vi "Read System Status.vi"(8 "error in (no error)":errorcluster) -> (0 "error out":errorcluster)   [LabVIEW 2018, in "cetoni.lvlib" / "cetoni.lvclass"]
uses:
  cetoni.lvclass
  Resources/GLOBAL/GLOBAL Time-critical.vi
  <userlib>/QmixLib/QmixLib.lvlib
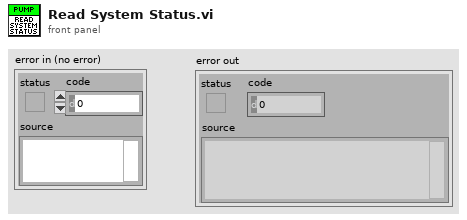
[diagram p1: front panel]
types:
  T1 = enum16{"LOW_PRESSURE_VALVE", "BALL_VALVE", "QMIX_VALVE"}
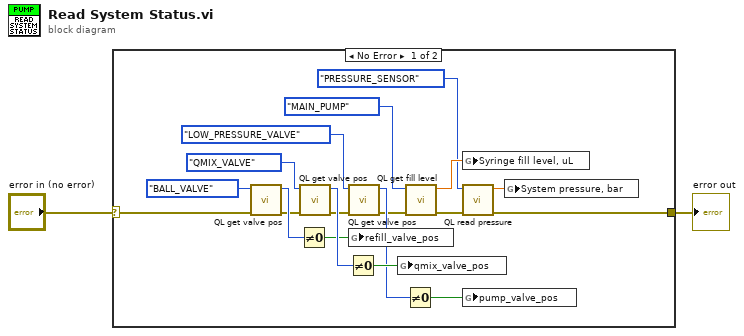
[diagram p0: block diagram]
diagram:
  n1 = case shown="No Error" "error in (no error)" {
    selector: "error in (no error)" -> [w12 w22]
    tunnel: [w5 w22] -> w1
    frame No Error {
      n2 = call <userlib>:"QL get valve pos.vi"("error in (no error) 2"=w12, "valve"=T1."BALL_VALVE") -> ("error out 2"=w11:errorcluster, "pos"=w14:i32)  [unwired: 8 in]
      n3 = Not Equal To 0?(x=w14) -> (x != 0?=w13:bool)
      n4 = call <userlib>:"QL get valve pos.vi"("error in (no error) 2"=w11, "valve"=T1."QMIX_VALVE") -> ("error out 2"=w10:errorcluster, "pos"=w19:i32)  [unwired: 8 in]
      n5 = Not Equal To 0?(x=w19) -> (x != 0?=w18:bool)
      n6 = call <userlib>:"QL get valve pos.vi"("error in (no error) 2"=w10, "valve"=T1."LOW_PRESSURE_VALVE") -> ("error out 2"=w9:errorcluster, "pos"=w16:i32)  [unwired: 8 in]
      n7 = global write "GLOBAL Time-critical.vi" "refill_valve_pos"(w13) -> ()
      n8 = global write "GLOBAL Time-critical.vi" "qmix_valve_pos"(w18) -> ()
      n9 = Not Equal To 0?(x=w16) -> (x != 0?=w15:bool)
      n10 = call <userlib>:"QL get fill level.vi"("error in (no error)"=w9, "pump"=enum16{"MAIN_PUMP"}."MAIN_PUMP") -> ("error out"=w4:errorcluster, "Fill level, uL"=w7:dbl)  [unwired: 8 in]
      n11 = global write "GLOBAL Time-critical.vi" "Syringe fill level, uL"(w7) -> ()
      n12 = call <userlib>:"QL read pressure.vi"("error in (no error)"=w4, "Pressure sensor"=enum16{"PRESSURE_SENSOR"}."PRESSURE_SENSOR") -> ("error out"=w5:errorcluster, "Pressure, bar"=w6:dbl)  [unwired: 8 in]
      n13 = global write "GLOBAL Time-critical.vi" "pump_valve_pos"(w15) -> ()
      n14 = global write "GLOBAL Time-critical.vi" "System pressure, bar"(w6) -> ()
    }
    frame Error {
    }
  }
  "error out" <- w1
